vi "NK11003_NK11003_CRC16.vi"(0 "input String":string) -> (1 "InPut +CRC":string, 2 "CRC16":string)   [LabVIEW 2015]
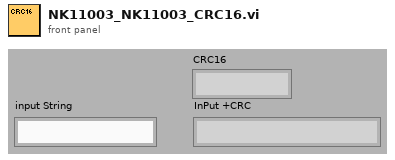
[diagram p1: front panel]
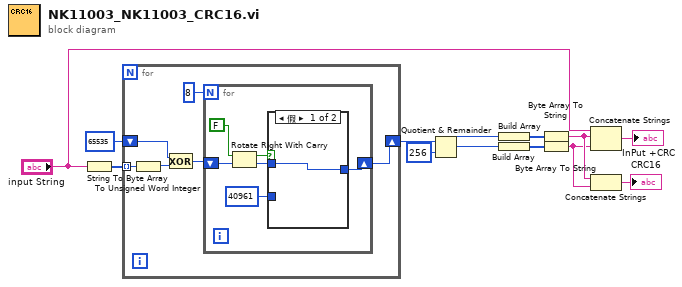
[diagram p0: block diagram]
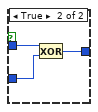
[diagram p2: hidden frame]
diagram:
  n1 = String To Byte Array(string="input String") -> (unsigned byte array=w13:u8[])
  n2 = for {
    tunnel: w13 -> [w19] mode=indexing
    shift-right: [w15] -> w7
    shift-left: 65535 -> [w17]
    n3 = To Unsigned Word Integer(number=w19) -> (unsigned 16bit integer=w18:u16)
    n4 = Exclusive Or(1:w18, 2:w17) -> (0:w16:i32)
    n5 = for {
      N: 8 -> [_]
      shift-right: [w20] -> w15
      shift-left: w16 -> [w25]
      n6 = Rotate Right With Carry(2:w25, 3:FALSE ("carry")) -> (0:w22:i32, 1:w23:bool)
      n7 = case shown="假" w23 {
        tunnel: w22 -> [w26 w29]
        tunnel: 40961 ("y") -> [_ w28]
        tunnel: [w26 w27] -> w20
        frame False {
        }
        frame True {
          n8 = Exclusive Or(1:w28, 2:w29) -> (0:w27:i32)
        }
      }
    }
  }
  n9 = Quotient & Remainder(x=w7, y=256) -> (x-y*floor(x/y)=w2:i32, floor(x/y)=w1:i32)
  n10 = Build Array(w2) -> (w11:i32[])
  n11 = Build Array(w1) -> (w10:i32[])
  n12 = Byte Array To String(unsigned byte array=w11) -> (string=w5:string)
  n13 = Byte Array To String(unsigned byte array=w10) -> (string=w4:string)
  n14 = Concatenate Strings("input String", w5, w4) -> (→"InPut +CRC":string)
  n15 = Concatenate Strings(w5, w4) -> (→"CRC16":string)
